vi "setErrorHandlingBehavior.vi"(8 "error in (no error)":errorcluster, 10 "Shutdown on Unhandled Error? (F)":bool, 11 "SMO in":refnum<class "SMO.lvclass">) -> (0 "error out":errorcluster, 3 "SMO out":refnum<class "SMO.lvclass">)   [LabVIEW 2021, in "smo.lvlib" / "SMO.lvclass"]
uses:
  SMO.lvclass
  SMO.lvclass/SMO.ctl
  Support/Attribute/Attribute.lvclass/Attribute.ctl
  Support/Attribute/Read AttrName.vi
  Private/ReftoDVR--SMO.vi
  Support/Attribute.ErrorHandling/Attribute.ErrorHandling.lvclass
  C:/Repositories/SMO/src/Support/Attribute/Attribute.lvclass
  <vilib>/Utility/LVClass/Get LV Class Name.vi
  <vilib>/Utility/error.llb/Error Cluster From Error Code.vi
  Support/Attribute/Attribute.lvclass
  C:/Repositories/SMO/src/Support/Attribute.ErrorHandling/Attribute.ErrorHandling.lvclass
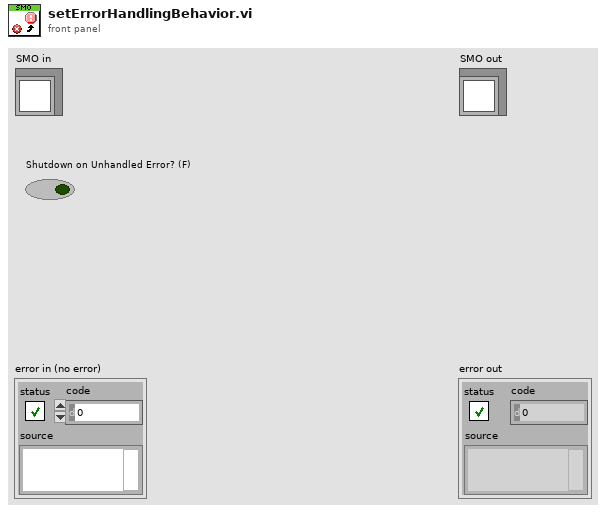
[diagram p1: front panel]
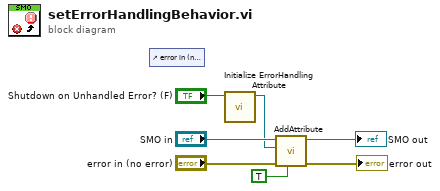
[diagram p0: block diagram]
diagram:
  n1 = control-ref of="error in (no error)"() -> ()  [unwired: 1 out]
  n2 = call "Initialize ErrorHandling Attribute.vi"("Shutdown on Unhandled Error"="Shutdown on Unhandled Error? (F)") -> ("Attribute.ErrorHandling"=w5:refnum<class "Attribute.ErrorHandling.lvclass">)  [unwired: 10 in]
  n3 = call "AddAttribute.vi"("Overwrite? (F)"=TRUE, "error in (no error)"="error in (no error)", "Attribute"=w5, "SMO in"="SMO in") -> ("error out"=→"error out":errorcluster, "SMO in"=→"SMO out":refnum<class "SMO.lvclass">)  [unwired: 6 in]
